vi "SetVariable.vi"(8 "error in":errorcluster, 9 "variable":string, 10 "value":dbl, 11 "lua_State *L":u64) -> (0 "error out":errorcluster)   [LabVIEW 2011]
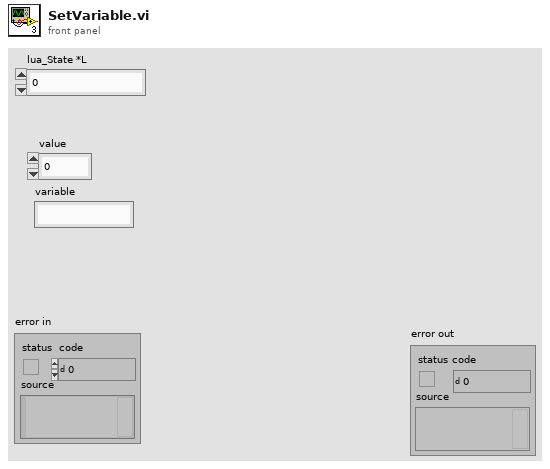
[diagram p1: front panel]
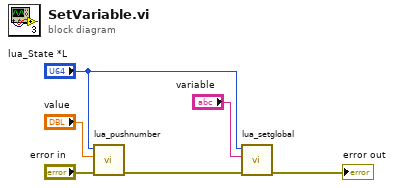
[diagram p0: block diagram]
diagram:
  n1 = call "lua_pushnumber.vi"("error in"="error in", "lua_Number n"="value", "lua_State *L"="lua_State *L") -> ("error out"=w5:errorcluster)  [unwired: 8 in]
  n2 = call "lua_setglobal.vi"("error in"=w5, "const char *k"="variable", "lua_State *L"="lua_State *L") -> ("error out"=→"error out":errorcluster)  [unwired: 8 in]
